vi "InitExpansionIO.vi"() -> (2 "AnalogIoObjects":T10, 3 "DigitalIoObjects":T26)   [LabVIEW 2014]
uses:
  <vilib>/Rock Robotics/WPI/MotorControl/WPI_MotorControlDeviceRef.ctl
  <vilib>/Rock Robotics/WPI/MotorControl/WPI_MotorControlType.ctl
  <vilib>/Rock Robotics/SystemInterfaces/Typedef/FPGA_TypedefDigitalModule.ctl
  <vilib>/Rock Robotics/SystemInterfaces/DIO/FPGA_DIOPWMChannel.ctl
  <vilib>/Rock Robotics/WPI/PWM/WPI_PWMDeadband.ctl
  <vilib>/Rock Robotics/WPI/CAN/Jaguar/SubVIs/WPI_CANJaguar_ControlMode.ctl
  <vilib>/Rock Robotics/WPI/CAN/TalonSRX/WPI_CANTalonSRX_APIControlMode.ctl
  <vilib>/Rock Robotics/WPI/PWM/WPI_PWMTransform_ConPane.ctl
  <vilib>/Rock Robotics/WPI/DigitalInput/WPI_DigitalInputDevRef.ctl
  <vilib>/Rock Robotics/SystemInterfaces/DIO/FPGA_DIOChannel.ctl
  <vilib>/Rock Robotics/WPI/DigitalOutput/WPI_DigitalOutputDevRef.ctl
  <vilib>/Rock Robotics/WPI/Encoder/WPI_EncoderDevRef.ctl
  <vilib>/Rock Robotics/SystemInterfaces/Encoder/FPGA_EncoderIdx.ctl
  <vilib>/Rock Robotics/SystemInterfaces/Counter/FPGA_CounterCtrSystemIndex.ctl
  <vilib>/Rock Robotics/WPI/Encoder/WPI_EncoderType.ctl
  <vilib>/Rock Robotics/WPI/AnalogChannel/WPI_AnalogChannelDevRef.ctl
  <vilib>/Rock Robotics/SystemInterfaces/Typedef/FPGA_TypedefAnalogModule.ctl
  <vilib>/Rock Robotics/SystemInterfaces/AI/FPGA_AIChannel.ctl
  <vilib>/Rock Robotics/SystemInterfaces/AnalogTrigger/FPGA_AnalogTriggerDevRef.ctl
  <vilib>/Rock Robotics/SystemInterfaces/AnalogTrigger/FPGA_AnalogTriggerIndex.ctl
  <vilib>/Rock Robotics/WPI/Counter/WPI_CounterDevRef.ctl
  <vilib>/Rock Robotics/WPI/AnalogOutput/WPI_AOChannelDevRef.ctl
  <vilib>/Rock Robotics/WPI/AnalogOutput/WPI_AnalogOutputChannel.ctl
  navX-MXP_PinTypeDef.ctl
  <vilib>/Rock Robotics/WPI/MotorControl/WPI_MotorControlOpen Victor.vi
  <vilib>/Rock Robotics/WPI/MotorControl/WPI_MotorControlOpen Jaguar.vi
  <vilib>/Rock Robotics/WPI/Counter/WPI_CounterDigitalInputToDigitalSource.vi
  <vilib>/Rock Robotics/WPI/Counter/WPI_CounterAnalogTriggerToDigitalSource.vi
  <vilib>/Rock Robotics/WPI/Counter/WPI_CounterOpen UpDown Mode.vi
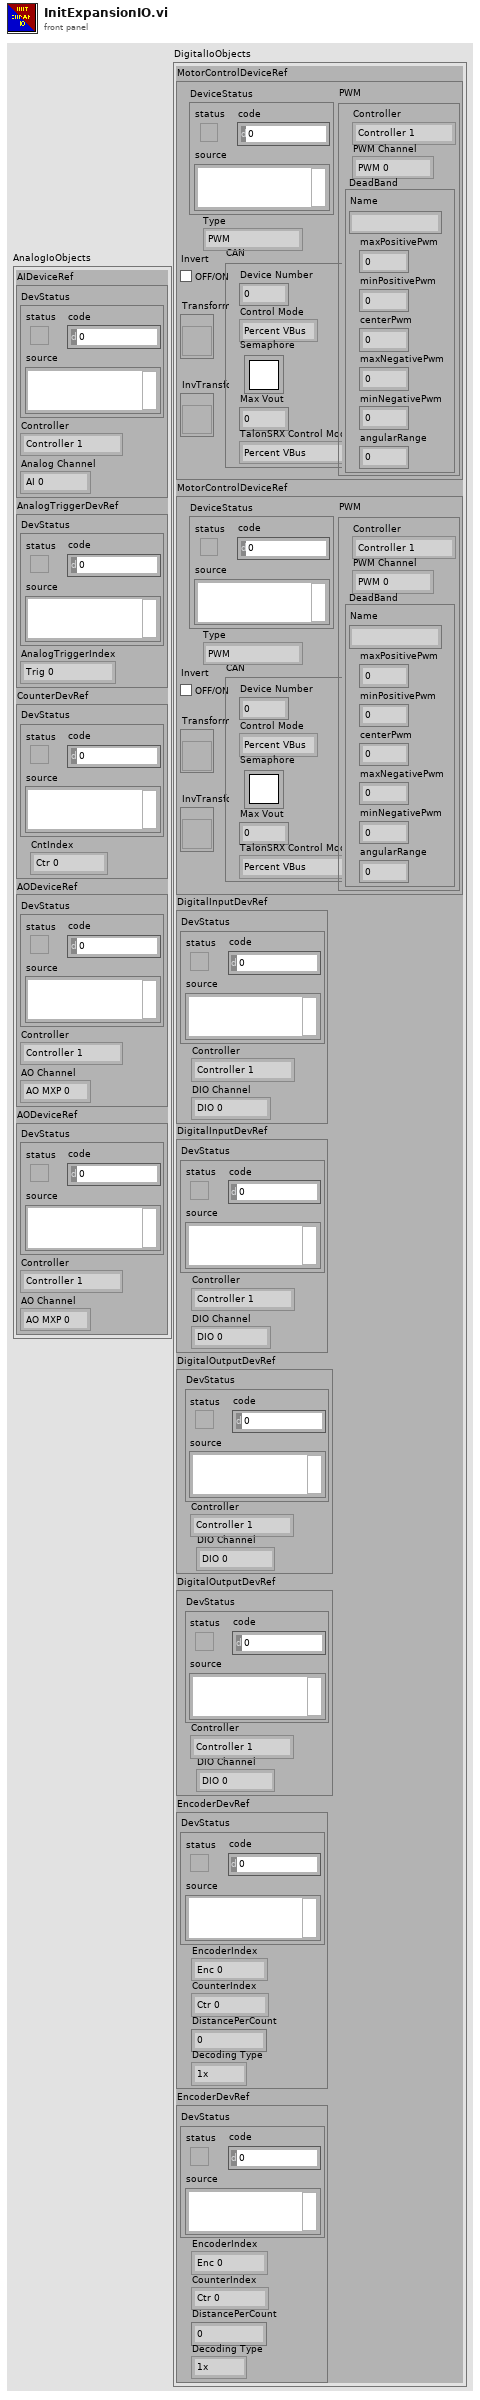
[diagram p1: front panel]
types:
  T1 = typedef "WPI_AnalogChannelDevRef.ctl" = cluster{"DevStatus":errorcluster, "Controller":T2, "Analog Channel":T3}
  T2 = typedef "FPGA_TypedefAnalogModule.ctl" = enum16{"Controller 1"}
  T3 = typedef "FPGA_AIChannel.ctl" = enum8{"AI 0", "AI 1", "AI 2", "AI 3", "AI MXP 0", "AI MXP 1", "AI MXP 2", "AI MXP 3", "Invalid"}
  T4 = typedef "FPGA_AnalogTriggerDevRef.ctl" = cluster{"DevStatus":errorcluster, "AnalogTriggerIndex":T5}
  T5 = typedef "FPGA_AnalogTriggerIndex.ctl" = enum8{"Trig 0", "Trig 1", "Trig 2", "Trig 3", "Trig 4", "Trig 5", "Trig 6", "Trig 7", "Invalid"}
  T6 = typedef "WPI_CounterDevRef.ctl" = cluster{"DevStatus":errorcluster, "CntIndex":T7}
  T7 = typedef "FPGA_CounterCtrSystemIndex.ctl" = enum8{"Ctr 0", "Ctr 1", "Ctr 2", "Ctr 3", "Ctr 4", "Ctr 5", "Ctr 6", "Ctr 7", "Invalid"}
  T8 = typedef "WPI_AOChannelDevRef.ctl" = cluster{"DevStatus":errorcluster, "Controller":T2, "AO Channel":T9}
  T9 = typedef "WPI_AnalogOutputChannel.ctl" = enum8{"AO MXP 0", "AO MXP 1", "Invalid"}
  T10 = cluster{"AIDeviceRef":T1, "AnalogTriggerDevRef":T4, "CounterDevRef":T6, "AODeviceRef":T8, "AODeviceRef":T8}
  T11 = typedef "WPI_MotorControlDeviceRef.ctl" = cluster{"DeviceStatus":errorcluster, "Type":T12, "PWM":cluster{"Controller":T13, "PWM Channel":T14, "DeadBand":T15}, "CAN":cluster{"Device Number":u8, "Control Mode":T16, "Semaphore":T17, "Max Vout":dbl, "TalonSRX Control Mode":T18}, "Invert":bool, "TransformRef":T19, "InvTransformRef":T19}
  T12 = typedef "WPI_MotorControlType.ctl" = enum16{"PWM", "CAN", "CANTalonSRX"}
  T13 = typedef "FPGA_TypedefDigitalModule.ctl" = enum16{"Controller 1"}
  T14 = typedef "FPGA_DIOPWMChannel.ctl" = enum8{"PWM 0", "PWM 1", "PWM 2", "PWM 3", "PWM 4", "PWM 5", "PWM 6", "PWM 7", "PWM 8", "PWM 9", "PWM MXP 0", "PWM MXP 1", "PWM MXP 2", "PWM MXP 3", "PWM MXP 4", "PWM MXP 5", "PWM MXP 6", "PWM MXP 7", "PWM MXP 8", "PWM MXP 9", "Invalid"}
  T15 = typedef "WPI_PWMDeadband.ctl" = cluster{"Name":string, "maxPositivePwm":i32, "minPositivePwm":i32, "centerPwm":i32, "maxNegativePwm":i32, "minNegativePwm":i32, "angularRange":u16}
  T16 = typedef "WPI_CANJaguar_ControlMode.ctl" = enum8{"Percent VBus", "Current", "Speed", "Position", "Voltage"}
  T17 = typedef "Semaphore RefNum" = refnum<k1>
  T18 = typedef "WPI_CANTalonSRX_APIControlMode.ctl" = enum8{"Percent VBus", "Speed", "Position", "Slave", "Unchanged / Invalid"}
  T19 = typedef "WPI_PWMTransform_ConPane.ctl" = refnum<vi>
  T20 = typedef "WPI_DigitalInputDevRef.ctl" = cluster{"DevStatus":errorcluster, "DIO Channel":T21, "Controller":T13}
  T21 = typedef "FPGA_DIOChannel.ctl" = enum8{"DIO 0", "DIO 1", "DIO 2", "DIO 3", "DIO 4", "DIO 5", "DIO 6", "DIO 7", "DIO 8", "DIO 9", "DIO MXP 0", "DIO MXP 1", "DIO MXP 2", "DIO MXP 3", "DIO MXP 4", "DIO MXP 5", "DIO MXP 6", "DIO MXP 7", "DIO MXP 8", "DIO MXP 9", "DIO MXP 10", "DIO MXP 11", "DIO MXP 12", "DIO MXP 13", "DIO MXP 14", "DIO MXP 15", "Invalid"}
  T22 = typedef "WPI_DigitalOutputDevRef.ctl" = cluster{"Controller":T13, "DIO Channel":T21, "DevStatus":errorcluster}
  T23 = typedef "WPI_EncoderDevRef.ctl" = cluster{"DevStatus":errorcluster, "EncoderIndex":T24, "CounterIndex":T7, "DistancePerCount":dbl, "Decoding Type":T25}
  T24 = typedef "FPGA_EncoderIdx.ctl" = enum8{"Enc 0", "Enc 1", "Enc 2", "Enc 3", "Enc 4", "Enc 5", "Enc 6", "Enc 7", "Invalid"}
  T25 = typedef "WPI_EncoderType.ctl" = enum16{"1x", "2x", "4x"}
  T26 = cluster{"MotorControlDeviceRef":T11, "MotorControlDeviceRef":T11, "DigitalInputDevRef":T20, "DigitalInputDevRef":T20, "DigitalOutputDevRef":T22, "DigitalOutputDevRef":T22, "EncoderDevRef":T23, "EncoderDevRef":T23}
  T27 = typedef "navX-MXP_PinTypeDef.ctl" = enum16{"DigitalIO", "PWM", "AnalogIn", "AnalogOut", ""}
  T28 = typedef "FPGA_CounterEncoderSourceConvertionLVSourceType.ctl" = cluster{"DevStatus":errorcluster, "AnalogTriggerMode?":bool, "DigitalMode":cluster{"Controller":T13, "DIO Channel":T29}, "AnalogTriggerMode":cluster{"AnalogTriggerIndex":T5, "OutputType":T30}}
  T29 = typedef "FPGA_DIODigitalSourceChannel.ctl" = enum8{"DIO 0", "DIO 1", "DIO 2", "DIO 3", "DIO 4", "DIO 5", "DIO 6", "DIO 7", "DIO 8", "DIO 9", "DIO MXP 0", "DIO MXP 1", "DIO MXP 2", "DIO MXP 3", "DIO MXP 4", "DIO MXP 5", "DIO MXP 6", "DIO MXP 7", "DIO MXP 8", "DIO MXP 9", "DIO MXP 10", "DIO MXP 11", "DIO MXP 12", "DIO MXP 13", "DIO MXP 14", "DIO MXP 15", "Disabled"}
  T30 = typedef "FPGA_AnalogTriggerOutType.ctl" = enum16{"InWindow", "TriggerState", "Rising", "Falling"}
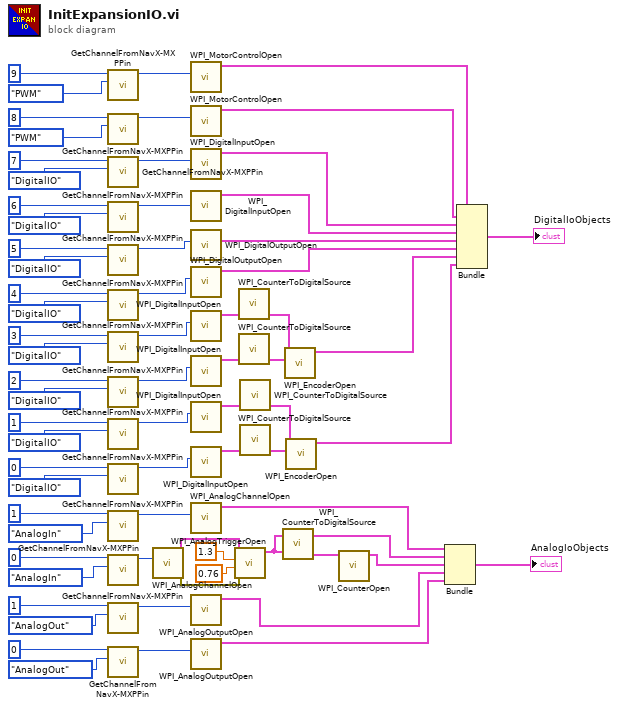
[diagram p0: block diagram]
diagram:
  n1 = call "GetChannelFromNavX-MXPPin.vi"("navX-MXP Pin Type"=navX-MXP_PinTypeDef."PWM" ("Enum"), "navX-MXP Pin Number"=9) -> ("RoboRIO Channel Number"=w54:u8)  [unwired: 9 in]
  n2 = call "GetChannelFromNavX-MXPPin.vi"("navX-MXP Pin Type"=navX-MXP_PinTypeDef."PWM" ("Enum"), "navX-MXP Pin Number"=8) -> ("RoboRIO Channel Number"=w53:u8)  [unwired: 9 in]
  n3 = call "GetChannelFromNavX-MXPPin.vi"("navX-MXP Pin Type"=navX-MXP_PinTypeDef."DigitalIO" ("Enum"), "navX-MXP Pin Number"=7) -> ("RoboRIO Channel Number"=w50:u8)  [unwired: 9 in]
  n4 = call "GetChannelFromNavX-MXPPin.vi"("navX-MXP Pin Type"=navX-MXP_PinTypeDef."DigitalIO" ("Enum"), "navX-MXP Pin Number"=6) -> ("RoboRIO Channel Number"=w47:u8)  [unwired: 9 in]
  n5 = call "GetChannelFromNavX-MXPPin.vi"("navX-MXP Pin Type"=navX-MXP_PinTypeDef."DigitalIO" ("Enum"), "navX-MXP Pin Number"=5) -> ("RoboRIO Channel Number"=w42:u8)  [unwired: 9 in]
  n6 = call "GetChannelFromNavX-MXPPin.vi"("navX-MXP Pin Type"=navX-MXP_PinTypeDef."DigitalIO" ("Enum"), "navX-MXP Pin Number"=4) -> ("RoboRIO Channel Number"=w41:u8)  [unwired: 9 in]
  n7 = call "GetChannelFromNavX-MXPPin.vi"("navX-MXP Pin Type"=navX-MXP_PinTypeDef."DigitalIO" ("Enum"), "navX-MXP Pin Number"=3) -> ("RoboRIO Channel Number"=w36:u8)  [unwired: 9 in]
  n8 = call "GetChannelFromNavX-MXPPin.vi"("navX-MXP Pin Type"=navX-MXP_PinTypeDef."DigitalIO" ("Enum"), "navX-MXP Pin Number"=2) -> ("RoboRIO Channel Number"=w35:u8)  [unwired: 9 in]
  n9 = call "GetChannelFromNavX-MXPPin.vi"("navX-MXP Pin Type"=navX-MXP_PinTypeDef."DigitalIO" ("Enum"), "navX-MXP Pin Number"=1) -> ("RoboRIO Channel Number"=w30:u8)  [unwired: 9 in]
  n10 = call "GetChannelFromNavX-MXPPin.vi"("navX-MXP Pin Type"=navX-MXP_PinTypeDef."DigitalIO" ("Enum"), "navX-MXP Pin Number"=0) -> ("RoboRIO Channel Number"=w29:u8)  [unwired: 9 in]
  n11 = call "GetChannelFromNavX-MXPPin.vi"("navX-MXP Pin Type"=navX-MXP_PinTypeDef."AnalogIn" ("Enum"), "navX-MXP Pin Number"=1) -> ("RoboRIO Channel Number"=w25:u8)  [unwired: 9 in]
  n12 = call "GetChannelFromNavX-MXPPin.vi"("navX-MXP Pin Type"=navX-MXP_PinTypeDef."AnalogIn" ("Enum"), "navX-MXP Pin Number"=0) -> ("RoboRIO Channel Number"=w13:u8)  [unwired: 9 in]
  n13 = call "GetChannelFromNavX-MXPPin.vi"("navX-MXP Pin Type"=navX-MXP_PinTypeDef."AnalogOut" ("Enum"), "navX-MXP Pin Number"=1) -> ("RoboRIO Channel Number"=w20:u8)  [unwired: 9 in]
  n14 = call "GetChannelFromNavX-MXPPin.vi"("navX-MXP Pin Type"=navX-MXP_PinTypeDef."AnalogOut" ("Enum"), "navX-MXP Pin Number"=0) -> ("RoboRIO Channel Number"=w17:u8)  [unwired: 9 in]
  n15 = call <vilib>:"WPI_AnalogChannelOpen.vi"("Analog Channel"=w13) -> ("error out"=w15:errorcluster, "AIDeviceRef"=w14:T1)  [unwired: 9 in]
  n16 = call-poly <vilib>:"WPI_MotorControlOpen.vi"("PWM Channel"=w54) -> ("MotorControlDeviceRef"=w70:T11)  [unwired: 9 in, 1 out]
  n17 = call-poly <vilib>:"WPI_MotorControlOpen.vi"("PWM Channel"=w53) -> ("MotorControlDeviceRef"=w56:T11)  [unwired: 9 in, 1 out]
  n18 = call <vilib>:"WPI_DigitalInputOpen.vi"("DIO Channel"=w50) -> ("DigitalInputDevRef"=w69:T20)  [unwired: 9 in, 1 out]
  n19 = call <vilib>:"WPI_DigitalInputOpen.vi"("DIO Channel"=w47) -> ("DigitalInputDevRef"=w68:T20)  [unwired: 9 in, 1 out]
  n20 = call <vilib>:"WPI_DigitalOutputOpen.vi"("DIO Channel"=w42) -> ("DigitalOutputDevRef"=w67:T22)  [unwired: 9 in, 1 out]
  n21 = call <vilib>:"WPI_DigitalOutputOpen.vi"("DIO Channel"=w41) -> ("DigitalOutputDevRef"=w55:T22)  [unwired: 9 in, 1 out]
  n22 = call <vilib>:"WPI_DigitalInputOpen.vi"("DIO Channel"=w36) -> ("DigitalInputDevRef"=w64:T20)  [unwired: 2 in, 8 out]
  n23 = call <vilib>:"WPI_DigitalInputOpen.vi"("DIO Channel"=w35) -> ("DigitalInputDevRef"=w65:T20)  [unwired: 2 in, 8 out]
  n24 = call <vilib>:"WPI_DigitalInputOpen.vi"("DIO Channel"=w30) -> ("DigitalInputDevRef"=w60:T20)  [unwired: 2 in, 8 out]
  n25 = call <vilib>:"WPI_DigitalInputOpen.vi"("DIO Channel"=w29) -> ("DigitalInputDevRef"=w61:T20)  [unwired: 2 in, 8 out]
  n26 = call <vilib>:"WPI_AnalogChannelOpen.vi"("Analog Channel"=w25) -> ("AIDeviceRef"=w10:T1)  [unwired: 9 in, 1 out]
  n27 = call <vilib>:"WPI_AnalogOutputOpen.vi"("AO Channel"=w20) -> ("AODeviceRef"=w7:T8)  [unwired: 9 in, 1 out]
  n28 = call <vilib>:"WPI_AnalogOutputOpen.vi"("AO Channel"=w17) -> ("AODeviceRef"=w6:T8)  [unwired: 9 in, 1 out]
  n29 = call <vilib>:"WPI_AnalogTriggerOpen.vi"("error in (no error)"=w15, "LowerLimit (v)"=0.76, "UpperLimit (v)"=1.3, "AnalogTriggerSource"=w14) -> ("AnalogTriggerDevRef"=w9:T4)  [unwired: 6 in, 1 out]
  n30 = call-poly <vilib>:"WPI_CounterToDigitalSource.vi"("DigitalInputDevRef"=w64) -> ("Digital Source"=w63:T28)  [unwired: 6 out]
  n31 = call-poly <vilib>:"WPI_CounterToDigitalSource.vi"("DigitalInputDevRef"=w65) -> ("Digital Source"=w66:T28)  [unwired: 6 out]
  n32 = call-poly <vilib>:"WPI_CounterToDigitalSource.vi"("DigitalInputDevRef"=w60) -> ("Digital Source"=w59:T28)  [unwired: 6 out]
  n33 = call-poly <vilib>:"WPI_CounterToDigitalSource.vi"("DigitalInputDevRef"=w61) -> ("Digital Source"=w62:T28)  [unwired: 6 out]
  n34 = call-poly <vilib>:"WPI_CounterToDigitalSource.vi"("AnalogTriggerDevRef"=w9) -> ("Digital Source"=w16:T28)  [unwired: 6 in]
  n35 = call <vilib>:"WPI_EncoderOpen.vi"("BSource"=w66, "ASource"=w63) -> ("EncoderDevRef"=w57:T23)  [unwired: 6 in, 3 out]
  n36 = call <vilib>:"WPI_EncoderOpen.vi"("BSource"=w62, "ASource"=w59) -> ("EncoderDevRef"=w58:T23)  [unwired: 6 in, 3 out]
  n37 = call-poly <vilib>:"WPI_CounterOpen.vi"("Up Source"=w16) -> ("CounterDevRef"=w8:T6)  [unwired: 6 in, 4 out]
  n38 = Bundle("AIDeviceRef"=w10, "AnalogTriggerDevRef"=w9, "CounterDevRef"=w8, "AODeviceRef"=w7, "AODeviceRef"=w6) -> (→"AnalogIoObjects":T10)  [unwired: 1 in]
  n39 = Bundle("MotorControlDeviceRef"=w70, "MotorControlDeviceRef"=w56, "DigitalInputDevRef"=w69, "DigitalInputDevRef"=w68, "DigitalOutputDevRef"=w67, "DigitalOutputDevRef"=w55, "EncoderDevRef"=w57, "EncoderDevRef"=w58) -> (→"DigitalIoObjects":T26)  [unwired: 1 in]
